vi "Version_2.0_Single_Column_Code.vi"() -> ()   [LabVIEW 2020] (continued)
            n10081 = call "Convert from Dynamic Data6"("Dynamic Data Type"=w10540) -> ("Array"=w10547:dbl[])  [unwired: 3 in]
            n10082 = call-poly <vilib>:"Append Waveforms.vi"("waveform B"=w10545, "waveform A"=w10546) -> ("waveform out"=w10544:waveform(dbl))  [unwired: 8 in, 1 out]
            n10083 = call "Convert from Dynamic Data7"("Dynamic Data Type"=w10544) -> ("Array"=w10548:dbl[])  [unwired: 3 in]
            n10084 = Bundle("Array"=w10547, "Array"=w10548) -> (→"Amplified Signal with Fluid Volume for SEC":cluster{"Array":dbl[], "Array":dbl[]})  [unwired: 1 in]
          }
        }
        n10085 = case shown="True" w10476 {
          tunnel: w10480 -> [w10524 w10531]
          tunnel: w10471 -> [_ w10530]
          tunnel: [w10523 w10529] -> w10478
          tunnel: w10479 -> [w10522 w10527]
          tunnel: [w10521 w10525] -> w10477
          tunnel: w10470 -> [_ w10526]
          frame False {
            n10086 = call-poly <vilib>:"Append Waveforms.vi"("waveform B"=waveform(dbl) {"t0"=timestamp(0 s since 1904-01-01), "dt"=1.0, "Y"=[]}, "waveform A"=w10522) -> ("waveform out"=w10521:waveform(dbl))  [unwired: 8 in, 1 out]
            n10087 = call-poly <vilib>:"Append Waveforms.vi"("waveform B"=waveform(dbl) {"t0"=timestamp(0 s since 1904-01-01), "dt"=1.0, "Y"=[]}, "waveform A"=w10524) -> ("waveform out"=w10523:waveform(dbl))  [unwired: 8 in, 1 out]
          }
          frame True {
            n10088 = call-poly <vilib>:"Append Waveforms.vi"("waveform B"=w10526, "waveform A"=w10527) -> ("waveform out"=w10525:waveform(dbl))  [unwired: 8 in, 1 out]
            n10089 = call "Convert from Dynamic Data10"("Dynamic Data Type"=w10525) -> ("Array"=w10532:dbl[])  [unwired: 3 in]
            n10090 = call-poly <vilib>:"Append Waveforms.vi"("waveform B"=w10530, "waveform A"=w10531) -> ("waveform out"=w10529:waveform(dbl))  [unwired: 8 in, 1 out]
            n10091 = call "Convert from Dynamic Data11"("Dynamic Data Type"=w10529) -> ("Array"=w10533:dbl[])  [unwired: 3 in]
            n10092 = Bundle("Array"=w10532, "Array"=w10533) -> (→"Amplified Signal with Fluid Volume Near Affinity Elution":cluster{"Array":dbl[], "Array":dbl[]})  [unwired: 1 in]
          }
        }
        n10093 = case shown="True" w10469 {
          tunnel: w10475 -> [w10509 w10516]
          tunnel: w10471 -> [_ w10515]
          tunnel: [w10508 w10514] -> w10473
          tunnel: w10474 -> [w10507 w10512]
          tunnel: [w10506 w10511] -> w10472
          tunnel: w10470 -> [_ w10510]
          frame False {
            n10094 = call-poly <vilib>:"Append Waveforms.vi"("waveform B"=waveform(dbl) {"t0"=timestamp(0 s since 1904-01-01), "dt"=1.0, "Y"=[]}, "waveform A"=w10507) -> ("waveform out"=w10506:waveform(dbl))  [unwired: 8 in, 1 out]
            n10095 = call-poly <vilib>:"Append Waveforms.vi"("waveform B"=waveform(dbl) {"t0"=timestamp(0 s since 1904-01-01), "dt"=1.0, "Y"=[]}, "waveform A"=w10509) -> ("waveform out"=w10508:waveform(dbl))  [unwired: 8 in, 1 out]
          }
          frame True {
            n10096 = call-poly <vilib>:"Append Waveforms.vi"("waveform B"=w10510, "waveform A"=w10512) -> ("waveform out"=w10511:waveform(dbl))  [unwired: 8 in, 1 out]
            n10097 = call "Convert from Dynamic Data8"("Dynamic Data Type"=w10511) -> ("Array"=w10517:dbl[])  [unwired: 3 in]
            n10098 = call-poly <vilib>:"Append Waveforms.vi"("waveform B"=w10515, "waveform A"=w10516) -> ("waveform out"=w10514:waveform(dbl))  [unwired: 8 in, 1 out]
            n10099 = call "Convert from Dynamic Data9"("Dynamic Data Type"=w10514) -> ("Array"=w10518:dbl[])  [unwired: 3 in]
            n10100 = Bundle("Array"=w10517, "Array"=w10518) -> (→"Amplified Signal with Fluid Volume for Affinity Elution":cluster{"Array":dbl[], "Array":dbl[]})  [unwired: 1 in]
          }
        }
        n10101 = call-poly <vilib>:"Append Waveforms.vi"("waveform B"=w10471, "waveform A"=w10503) -> ("waveform out"=w10496:waveform(dbl))  [unwired: 8 in, 1 out]
        n10102 = call "Convert from Dynamic Data3"("Dynamic Data Type"=w10496) -> ("Array"=w10499:dbl[])  [unwired: 3 in]
        n10103 = Bundle("Array"=w10498, "Array"=w10499) -> (→"Amplified Signal with Fluid Volume":cluster{"Array":dbl[], "Array":dbl[]})  [unwired: 1 in]
        n10104 = Wait Until Next ms Multiple(millisecond multiple=u32 400) -> ()  [unwired: 1 out]
      }
      n10105 = call-poly "VISA Configure Serial Port"("VISA resource name"=refnum<visa-resource-name> "COM7", "timeout (10sec)"=u32 1000, "baud rate (9600)"=u32 9600) -> ("VISA resource name out"=w69:refnum<visa-resource-name>, "error out"=w68:errorcluster)  [unwired: 11 in]
      n10106 = call <vilib>:"fgt init.vi"() -> ("error out"=w28:errorcluster)  [unwired: 11 in]
      n10107 = call <vilib>:"fgt init.vi"() -> ("error out"=w18:errorcluster)  [unwired: 11 in]
      n10108 = call <vilib>:"fgt init.vi"() -> ("error out"=w12:errorcluster)  [unwired: 11 in]
      n10109 = call <vilib>:"fgt init.vi"() -> ("error out"=w14:errorcluster)  [unwired: 11 in]
      n10110 = call <vilib>:"fgt init.vi"() -> ("error out"=w20:errorcluster)  [unwired: 11 in]
      n10111 = call <vilib>:"fgt init.vi"() -> ("error out"=w16:errorcluster)  [unwired: 11 in]
      n10112 = call <vilib>:"fgt init.vi"() -> ("error out"=w22:errorcluster)  [unwired: 11 in]
      n10113 = call <vilib>:"fgt init.vi"() -> ("error out"=w26:errorcluster)  [unwired: 11 in]
      n10114 = call <vilib>:"fgt init.vi"() -> ("error out"=w24:errorcluster)  [unwired: 11 in]
      n10115 = while {
        tunnel: w28 -> [w478]
        tunnel: [w477] -> w27
        tunnel: w26 -> [w476]
        tunnel: [w475] -> w25
        tunnel: w24 -> [w474]
        tunnel: [w473] -> w23
        tunnel: w22 -> [w472]
        tunnel: [w471] -> w21
        tunnel: w20 -> [w470]
        tunnel: [w469] -> w19
        tunnel: w18 -> [w468]
        tunnel: [w467] -> w17
        tunnel: w16 -> [w466]
        tunnel: [w465] -> w15
        tunnel: w14 -> [w464]
        tunnel: [w463] -> w13
        tunnel: w12 -> [w462]
        tunnel: [w461] -> w11
        stop <- w488 stop-if-true
        # "- Controls the 7 on-chip Valves. \n- By default pressure is applied to close them\n- On-chip Valve opening pressure is applied same as the \nsuction pressure for grid deposition on all the valves"
        n10116 = local read "Valve V1 Open"() -> (w508:bool)
        n10117 = local read "Valve V2 Open"() -> (w494:bool)
        n10118 = local read "Valve V3 Open"() -> (w493:bool)
        n10119 = local read "Valve V4 Open"() -> (w492:bool)
        n10120 = local read "Valve V5 Open"() -> (w491:bool)
        n10121 = local read "Valve V6 Open"() -> (w490:bool)
        n10122 = local read "Valve V7 Open"() -> (w489:bool)
        n10123 = Wait (ms)(milliseconds to wait=u32 100) -> ()  [unwired: 1 out]
        n10124 = local read "Valve V8 Open"() -> (w483:bool)
        n10125 = local read "On-Chip Valve \nClosing\nPressure (mbar)"() -> (w486:dbl)
        n10126 = local read "Stopper that ends \nthe main loops"() -> (w488:bool)
        n10127 = case shown="True" w508 {
          tunnel: [1 0 ("position")] -> w507
          frame False {
          }
          frame True {
          }
        }
        n10128 = case shown="True" w494 {
          tunnel: [1 0 ("position")] -> w505
          frame False {
          }
          frame True {
          }
        }
        n10129 = case shown="True" w493 {
          tunnel: [1 0 ("position")] -> w504
          frame False {
          }
          frame True {
          }
        }
        n10130 = case shown="True" w492 {
          tunnel: [1 0 ("position")] -> w501
          frame False {
          }
          frame True {
          }
        }
        n10131 = case shown="True" w491 {
          tunnel: [1 0 ("position")] -> w499
          frame False {
          }
          frame True {
          }
        }
        n10132 = case shown="True" w490 {
          tunnel: [1 0 ("position")] -> w497
          frame False {
          }
          frame True {
          }
        }
        n10133 = call <vilib>:"fgt set pressure.vi"("error in (no error)"=w478, "pressure"=w486, "pressureIndex"=0 ("module")) -> ("error out"=w477:errorcluster)  [unwired: 8 in]
        n10134 = call <vilib>:"fgt get pressure.vi"("pressureIndex"=u32 1) -> ("pressure out"=w481:sgl)  [unwired: 9 in, 1 out]
        n10135 = call <vilib>:"fgt get pressure.vi"("pressureIndex"=u32 0) -> ("pressure out"=w479:sgl)  [unwired: 9 in, 1 out]
        n10136 = case shown="True" w489 {
          tunnel: [1 0 ("position")] -> w495
          frame False {
          }
          frame True {
          }
        }
        n10137 = case shown="True" w483 {
          tunnel: [1 0 ("position")] -> w484
          frame False {
          }
          frame True {
          }
        }
        n10138 = call <vilib>:"fgt set valve position.vi"("error in (no error)"=w462, "position"=w507, "valveIndex"=u32 0) -> ("error out"=w461:errorcluster)  [unwired: 8 in]
        n10139 = call <vilib>:"fgt set valve position.vi"("error in (no error)"=w464, "position"=w505, "valveIndex"=u32 1) -> ("error out"=w463:errorcluster)  [unwired: 8 in]
        n10140 = call <vilib>:"fgt set valve position.vi"("error in (no error)"=w466, "position"=w504, "valveIndex"=u32 2) -> ("error out"=w465:errorcluster)  [unwired: 8 in]
        n10141 = call <vilib>:"fgt set valve position.vi"("error in (no error)"=w468, "position"=w501, "valveIndex"=u32 3) -> ("error out"=w467:errorcluster)  [unwired: 8 in]
        n10142 = call <vilib>:"fgt set valve position.vi"("error in (no error)"=w470, "position"=w499, "valveIndex"=u32 4) -> ("error out"=w469:errorcluster)  [unwired: 8 in]
        n10143 = call <vilib>:"fgt set valve position.vi"("error in (no error)"=w472, "position"=w497, "valveIndex"=u32 5) -> ("error out"=w471:errorcluster)  [unwired: 8 in]
        n10144 = local write "Valve Closing \nPressure Measured"(w479) -> ()
        n10145 = call <vilib>:"fgt set valve position.vi"("error in (no error)"=w474, "position"=w495, "valveIndex"=u32 6) -> ("error out"=w473:errorcluster)  [unwired: 8 in]
        n10146 = call <vilib>:"fgt set valve position.vi"("error in (no error)"=w476, "position"=w484, "valveIndex"=u32 7) -> ("error out"=w475:errorcluster)  [unwired: 8 in]
        n10147 = local write "Suction pressure \nmeasured"(w481) -> ()
      }
      n10148 = call <vilib>:"fgt close.vi"("error in (no error)"=w27) -> ()  [unwired: 10 in, 1 out]
      n10149 = call <vilib>:"fgt close.vi"("error in (no error)"=w17) -> ()  [unwired: 10 in, 1 out]
      n10150 = call <vilib>:"fgt close.vi"("error in (no error)"=w11) -> ()  [unwired: 10 in, 1 out]
      n10151 = call <vilib>:"fgt close.vi"("error in (no error)"=w13) -> ()  [unwired: 10 in, 1 out]
      n10152 = call <vilib>:"fgt close.vi"("error in (no error)"=w19) -> ()  [unwired: 10 in, 1 out]
      n10153 = call <vilib>:"fgt close.vi"("error in (no error)"=w15) -> ()  [unwired: 10 in, 1 out]
      n10154 = call <vilib>:"fgt close.vi"("error in (no error)"=w21) -> ()  [unwired: 10 in, 1 out]
      n10155 = call <vilib>:"fgt close.vi"("error in (no error)"=w25) -> ()  [unwired: 10 in, 1 out]
      n10156 = call <vilib>:"fgt close.vi"("error in (no error)"=w23) -> ()  [unwired: 10 in, 1 out]
      n10157 = while {
        stop <- w98 stop-if-true
        n10158 = event shown="[2] \"Stop for End of  Experiment  and Data Writing\": Value Change" {
          selector: _ -> [_ _ _]
          dyn-events: _ -> [_ _ _]
          timeout: 100 -> [_ _ _]
          tunnel: [_ _ w105] -> w98
          event Timeout {
            n10159 = event-data() -> ()  [unwired: 1 in, 3 out]
          }
          event "External Valve \nOpen": Value Change {
            n10160 = event-data() -> ()  [unwired: 1 in, 6 out]
            n10161 = local read "External Valve \nOpen"() -> (w100:bool)
            n10162 = case shown="False" w100 {
              frame False {
                # "external vale is closed"
                n10163 = local read "VISA Refnum in\nfor Valve"() -> (w102:refnum<visa-resource-name>)
                n10164 = call "PortChanger_Valve (SubVI).vi"("Port Number"="2", "VISA Refnum in"=w102) -> ()  [unwired: 10 in]
              }
              frame True {
                # "External valve is open"
                n10165 = local read "VISA Refnum in\nfor Valve"() -> (w104:refnum<visa-resource-name>)
                n10166 = call "PortChanger_Valve (SubVI).vi"("Port Number"="1", "VISA Refnum in"=w104) -> ()  [unwired: 10 in]
              }
            }
          }
          event "Stop for End of \nExperiment \nand Data Writing": Value Change {
            n10167 = event-data() -> ()  [unwired: 1 in, 6 out]
            n10168 = local read "Stop for End of \nExperiment \nand Data Writing"() -> (w105:bool)
          }
        }
      }
      n10169 = while {
        tunnel: [w120] -> w71
        tunnel: [w122] -> w70
        tunnel: w69 -> [w133]
        tunnel: w68 -> [w132]
        shift-right: [w121] -> _
        shift-left: w72 -> [w131]
        tunnel: [w130] -> w83
        tunnel: [w129] -> w84
        tunnel: w85 -> [w114]
        tunnel: [w114] -> w86
        tunnel: w10 -> [w112]
        tunnel: w9 -> [w113]
        stop <- w115 stop-if-true
        n10170 = local write "Position"(0 ("Position")) -> ()
        n10171 = local write "k1"(0.0 ("k1")) -> ()
        n10172 = local write "k2"(0.0 ("k2")) -> ()
        n10173 = event shown="[0] \"Select the Action\": Value Change" {
          selector: _ -> [_ _ _ _ _ _ _ _ _ _]
          dyn-events: _ -> [_ _ _ _ _ _ _ _ _ _]
          timeout: 100 -> [_ _ _ _ _ _ _ _ _ _]
          tunnel: w133 -> [w160 w410 w420 w431 w434 w439 w444 w449 w453 w460]
          tunnel: w132 -> [w159 w409 w419 w430 w435 w440 w445 w450 w452 w459]
          tunnel: w131 -> [_ _ _ _ _ _ _ _ _ _]
          tunnel: w112 -> [_ _ _ _ _ _ _ _ w455 w458]
          tunnel: w113 -> [_ _ _ _ _ _ _ _ w454 w457]
          tunnel: [w156 w407 w417 w427 _ _ _ _ w454 w457] -> w130
          tunnel: [w155 _ _ _ _ _ _ _ w455 w458] -> w129
          tunnel: [_ _ _ _ _ _ _ _ w456 _] -> w115
          tunnel: [w158 w408 w418 w428 w432 w437 w442 w447 w453 w460] -> w124
          tunnel: [w157 _ _ _ w433 w438 w443 w448 w452 w459] -> w123
          tunnel: w112 -> [w152 _ _ _ _ _ _ _ _ _]
          tunnel: w113 -> [w153 _ _ _ _ _ _ _ _ _]
          event "Select the Action": Value Change {
            n10174 = event-data() -> ()  [unwired: 1 in, 6 out]
            n10175 = local read "Select the Action"() -> (w154:T1)
            n10176 = case shown="\"Spread the deposited protein on the grid in One Line and plunge\"" w154 {
              tunnel: [w167 w174 w182 w266 w289 w377] -> w158
              tunnel: [w166 w173 w181 w265 w288 w376] -> w157
              tunnel: w160 -> [w165 w172 w180 w270 w287 w375]
              tunnel: w159 -> [w164 w171 w179 w269 w286 w374]
              tunnel: w152 -> [w161 w168 w178 w267 w285 w373]
              tunnel: w153 -> [w162 w169 w177 w268 w284 w372]
              tunnel: [w162 w169 w175 w268 w282 w372] -> w156
              tunnel: [w161 w168 w176 w267 w283 w373] -> w155
              frame .."Turn off Stepper Motor" {
                n10177 = VISA Write(VISA resource name=w165, write buffer="f", error in (no error)=w164) -> (VISA resource name out=w167:refnum<visa-resource-name>, error out=w166:errorcluster)  [unwired: 1 out]
              }
              frame "Turn  on Stepper Motor" {
                n10178 = VISA Write(VISA resource name=w172, write buffer="n", error in (no error)=w171) -> (VISA resource name out=w174:refnum<visa-resource-name>, error out=w173:errorcluster)  [unwired: 1 out]
              }
              frame "Start Plunging" {
                n10179 = stacked-sequence {
                  seq-local: [_ _ _ _ _ w204 _] -> [_ _ _ _ _ _ w263]
                  seq-local: [_ _ _ _ _ w203 _] -> [_ _ _ _ _ _ w262]
                  seq-local: [w184 _ _ _ _ _ _] -> [_ w191 _ _ _ _ _]
                  seq-local: [w183 _ _ _ _ _ _] -> [_ w190 _ _ _ _ _]
                  seq-local: [_ w189 _ _ _ _ _] -> [_ _ _ _ _ w202 _]
                  seq-local: [_ w188 _ _ _ _ _] -> [_ _ _ _ _ w201 _]
                  tunnel: [_ _ _ _ _ _ w261] -> w182
                  tunnel: [_ _ _ _ _ _ w260] -> w181
                  tunnel: w180 -> [_ _ _ _ _ w206 _]
                  tunnel: w179 -> [_ _ _ _ _ w205 _]
                  tunnel: w178 -> [w185 _ _ _ _ _ _]
                  tunnel: w177 -> [w186 _ _ _ _ _ _]
                  tunnel: [_ _ _ _ _ w200 _] -> w176
                  tunnel: [_ _ _ _ _ w199 _] -> w175
                  frame #0 {
                    w187 = 1 items=["Channel1"=1, "Channel2"=2, "Channel3"=3, "Channel4"=4] ("channel")
                    n10180 = invoke class="KCubeInertialMotor" method="SetPositionToZero"(reference=w185, error in=w186, "channel"=w187) -> (reference out=w184:refnum<k24>, error out=w183:errorcluster)  [unwired: 1 in, 2 out]
                  }
                  frame #1 {
                    w192 = 2 items=["Channel1"=1, "Channel2"=2, "Channel3"=3, "Channel4"=4] ("channel")
                    n10181 = invoke class="KCubeInertialMotor" method="SetPositionToZero"(reference=w191, error in=w190, "channel"=w192) -> (reference out=w189:refnum<k24>, error out=w188:errorcluster)  [unwired: 1 in, 2 out]
                  }
                  frame #2 {
                    n10182 = local write "Re-deposit Sample\nonto Grid"(FALSE ("Re-deposit Sample\nonto Grid")) -> ()
                    n10183 = local write "Divert Sample \nonto Grid"(TRUE ("Divert Sample \nonto Grid")) -> ()
                    n10184 = local read "Grid Deposition\nDuration"() -> (w193:u32)
                    n10185 = Wait (ms)(milliseconds to wait=w193) -> ()  [unwired: 1 out]
                  }
                  frame #3 {
                    n10186 = local write "Suction On/Off"(TRUE ("Suction On/Off")) -> ()
                  }
                  frame #4 {
                    n10187 = local read "Delay before\n1st movement\nof grid"() -> (w197:dbl)
                    n10188 = Wait (ms)(milliseconds to wait=w197) -> ()  [unwired: 1 out]
                  }
                  frame #5 {
                    n10189 = local read "No of cycles\nof up-down\nmovement"() -> (w198:dbl)
                    n10190 = for {
                      N: w198 -> [_]
                      shift-right: [w212] -> w204
                      shift-left: w206 -> [w214]
                      shift-right: [w211] -> w203
                      shift-left: w205 -> [w213]
                      shift-right: [w208] -> w200
                      shift-left: w202 -> [w210]
                      shift-right: [w207] -> w199
                      shift-left: w201 -> [w209]
                      n10191 = stacked-sequence {
                        seq-local: [w216 _ _ _ _ _] -> [_ _ _ w238 _ _]
                        seq-local: [w215 _ _ _ _ _] -> [_ _ _ w237 _ _]
                        seq-local: [_ _ w222 _ _ _] -> [_ _ _ _ _ w246]
                        seq-local: [_ _ w221 _ _ _] -> [_ _ _ _ _ w245]
                        tunnel: [_ _ _ w239 _ _] -> w212
                        tunnel: [_ _ _ w241 _ _] -> w211
                        tunnel: w214 -> [w219 _ _ _ _ _]
                        tunnel: w213 -> [w218 _ _ _ _ _]
                        tunnel: w210 -> [_ _ w224 _ _ _]
                        tunnel: w209 -> [_ _ w223 _ _ _]
                        tunnel: [_ _ _ _ _ w244] -> w208
                        tunnel: [_ _ _ _ _ w243] -> w207
                        frame #0 {
                          n10192 = VISA Write(VISA resource name=w219, write buffer="d", error in (no error)=w218) -> (VISA resource name out=w216:refnum<visa-resource-name>, error out=w215:errorcluster)  [unwired: 1 out]
                        }
                        frame #1 {
                          n10193 = local read "Duration for \nup/down\nMovement of Grid"() -> (w220:u32)
                          n10194 = Wait (ms)(milliseconds to wait=w220) -> ()  [unwired: 1 out]
                        }
                        frame #2 {
                          n10195 = stacked-sequence {
                            tunnel: w224 -> [_ w232 _]
                            tunnel: w223 -> [_ w231 _]
                            tunnel: [_ w230 _] -> w222
                            tunnel: [_ w229 _] -> w221
                            frame #0 {
                              n10196 = local read "Translation Step SIze\nwhile plunging"() -> (w225:dbl)
                              n10197 = local read "k1"() -> (w227:dbl)
                              n10198 = Decrement(x=w227) -> (x-1=w226:dbl)
                              n10199 = Multiply(x=w225, y=w226) -> (x*y=w228:dbl)
                              n10200 = local write "k2"(w226) -> ()
                              n10201 = local write "Position"(w228) -> ()
                            }
                            frame #1 {
                              w235 = 1 items=["Channel1"=1, "Channel2"=2, "Channel3"=3, "Channel4"=4] ("channel")
                              n10202 = local read "Position"() -> (w234:i32)
                              n10203 = invoke class="KCubeInertialMotor" method="MoveTo"(reference=w232, error in=w231, "channel"=w235, "position"=w234, "waitTimeout"=10000) -> (reference out=w230:refnum<k24>, error out=w229:errorcluster)  [unwired: 1 in, 4 out]
                            }
                            frame #2 {
                              n10204 = local read "Wait time for\ntranslation"() -> (w236:u32)
                              n10205 = Wait (ms)(milliseconds to wait=w236) -> ()  [unwired: 1 out]
                            }
                          }
                        }
                        frame #3 {
                          n10206 = VISA Write(VISA resource name=w238, write buffer="u", error in (no error)=w237) -> (VISA resource name out=w239:refnum<visa-resource-name>, error out=w241:errorcluster)  [unwired: 1 out]
                        }
                        frame #4 {
                          n10207 = local read "Duration for \nup/down\nMovement of Grid"() -> (w242:u32)
                          n10208 = Wait (ms)(milliseconds to wait=w242) -> ()  [unwired: 1 out]
                        }
                        frame #5 {
                          n10209 = stacked-sequence {
                            tunnel: w246 -> [_ w254 _]
                            tunnel: w245 -> [_ w253 _]
                            tunnel: [_ w252 _] -> w244
                            tunnel: [_ w251 _] -> w243
                            frame #0 {
                              n10210 = local read "Translation Step SIze\nwhile plunging"() -> (w247:dbl)
                              n10211 = local read "k2"() -> (w249:dbl)
                              n10212 = Increment(x=w249) -> (x+1=w248:dbl)
                              n10213 = Multiply(x=w247, y=w248) -> (x*y=w250:dbl)
                              n10214 = local write "k1"(w248) -> ()
                              n10215 = local write "Position"(w250) -> ()
                            }
                            frame #1 {
                              w257 = 1 items=["Channel1"=1, "Channel2"=2, "Channel3"=3, "Channel4"=4] ("channel")
                              n10216 = local read "Position"() -> (w256:i32)
                              n10217 = invoke class="KCubeInertialMotor" method="MoveTo"(reference=w254, error in=w253, "channel"=w257, "position"=w256, "waitTimeout"=10000) -> (reference out=w252:refnum<k24>, error out=w251:errorcluster)  [unwired: 1 in, 4 out]
                            }
                            frame #2 {
                              n10218 = local read "Wait time for\ntranslation"() -> (w258:u32)
                              n10219 = Wait (ms)(milliseconds to wait=w258) -> ()  [unwired: 1 out]
                            }
                          }
                        }
                      }
                    }
                  }
                  frame #6 {
                    n10220 = VISA Write(VISA resource name=w263, write buffer="p", error in (no error)=w262) -> (VISA resource name out=w261:refnum<visa-resource-name>, error out=w260:errorcluster)  [unwired: 1 out]
                    n10221 = local write "Suction On/Off"(FALSE ("Suction On/Off")) -> ()
                  }
                }
              }
              frame "Reset Plunger" {
                n10222 = stacked-sequence {
                  seq-local: [w272 _] -> [_ w280]
                  seq-local: [w271 _] -> [_ w279]
                  tunnel: w270 -> [w276 _]
                  tunnel: w269 -> [w275 _]
                  tunnel: [_ w278] -> w266
                  tunnel: [_ w277] -> w265
                  frame #0 {
                    n10223 = VISA Write(VISA resource name=w276, write buffer="r", error in (no error)=w275) -> (VISA resource name out=w272:refnum<visa-resource-name>, error out=w271:errorcluster)  [unwired: 1 out]
                    n10224 = Wait (ms)(milliseconds to wait=u32 1000) -> ()  [unwired: 1 out]
                  }
                  frame #1 {
                    n10225 = VISA Write(VISA resource name=w280, write buffer="f", error in (no error)=w279) -> (VISA resource name out=w278:refnum<visa-resource-name>, error out=w277:errorcluster)  [unwired: 1 out]
                  }
                }
              }
              frame "Spread the deposited protein on the grid and plunge" {
                n10226 = stacked-sequence {
                  seq-local: [_ _ _ _ _ w311 _] -> [_ _ _ _ _ _ w370]
                  seq-local: [_ _ _ _ _ w310 _] -> [_ _ _ _ _ _ w369]
                  seq-local: [w291 _ _ _ _ _ _] -> [_ w298 _ _ _ _ _]
                  seq-local: [w290 _ _ _ _ _ _] -> [_ w297 _ _ _ _ _]
                  seq-local: [_ w296 _ _ _ _ _] -> [_ _ _ _ _ w309 _]
                  seq-local: [_ w295 _ _ _ _ _] -> [_ _ _ _ _ w308 _]
                  tunnel: [_ _ _ _ _ _ w368] -> w289
                  tunnel: [_ _ _ _ _ _ w367] -> w288
                  tunnel: w287 -> [_ _ _ _ _ w313 _]
                  tunnel: w286 -> [_ _ _ _ _ w312 _]
                  tunnel: w285 -> [w292 _ _ _ _ _ _]
                  tunnel: w284 -> [w293 _ _ _ _ _ _]
                  tunnel: [_ _ _ _ _ w307 _] -> w283
                  tunnel: [_ _ _ _ _ w306 _] -> w282
                  frame #0 {
                    w294 = 1 items=["Channel1"=1, "Channel2"=2, "Channel3"=3, "Channel4"=4] ("channel")
                    n10227 = invoke class="KCubeInertialMotor" method="SetPositionToZero"(reference=w292, error in=w293, "channel"=w294) -> (reference out=w291:refnum<k24>, error out=w290:errorcluster)  [unwired: 1 in, 2 out]
                  }
                  frame #1 {
                    w299 = 2 items=["Channel1"=1, "Channel2"=2, "Channel3"=3, "Channel4"=4] ("channel")
                    n10228 = invoke class="KCubeInertialMotor" method="SetPositionToZero"(reference=w298, error in=w297, "channel"=w299) -> (reference out=w296:refnum<k24>, error out=w295:errorcluster)  [unwired: 1 in, 2 out]
                  }
                  frame #2 {
                    n10229 = local write "Re-deposit Sample\nonto Grid"(FALSE ("Re-deposit Sample\nonto Grid")) -> ()
                    n10230 = local write "Divert Sample \nonto Grid"(TRUE ("Divert Sample \nonto Grid")) -> ()
                    n10231 = local read "Grid Deposition\nDuration"() -> (w300:u32)
                    n10232 = Wait (ms)(milliseconds to wait=w300) -> ()  [unwired: 1 out]
                  }
                  frame #3 {
                    n10233 = local write "Suction On/Off"(TRUE ("Suction On/Off")) -> ()
                  }
                  frame #4 {
                    n10234 = local read "Delay before\n1st movement\nof grid"() -> (w304:dbl)
                    n10235 = Wait (ms)(milliseconds to wait=w304) -> ()  [unwired: 1 out]
                  }
                  frame #5 {
                    n10236 = local read "No of cycles\nof up-down\nmovement"() -> (w305:dbl)
                    n10237 = for {
                      N: w305 -> [_]
                      shift-right: [w319] -> w311
                      shift-left: w313 -> [w321]
                      shift-right: [w318] -> w310
                      shift-left: w312 -> [w320]
                      shift-right: [w315] -> w307
                      shift-left: w309 -> [w317]
                      shift-right: [w314] -> w306
                      shift-left: w308 -> [w316]
                      n10238 = stacked-sequence {
                        seq-local: [w323 _ _ _ _ _] -> [_ _ _ w345 _ _]
                        seq-local: [w322 _ _ _ _ _] -> [_ _ _ w344 _ _]
                        seq-local: [_ _ w329 _ _ _] -> [_ _ _ _ _ w353]
                        seq-local: [_ _ w328 _ _ _] -> [_ _ _ _ _ w352]
                        tunnel: [_ _ _ w346 _ _] -> w319
                        tunnel: [_ _ _ w348 _ _] -> w318
                        tunnel: w321 -> [w326 _ _ _ _ _]
                        tunnel: w320 -> [w325 _ _ _ _ _]
                        tunnel: w317 -> [_ _ w331 _ _ _]
                        tunnel: w316 -> [_ _ w330 _ _ _]
                        tunnel: [_ _ _ _ _ w351] -> w315
                        tunnel: [_ _ _ _ _ w350] -> w314
                        frame #0 {
                          n10239 = VISA Write(VISA resource name=w326, write buffer="d", error in (no error)=w325) -> (VISA resource name out=w323:refnum<visa-resource-name>, error out=w322:errorcluster)  [unwired: 1 out]
                        }
                        frame #1 {
                          n10240 = local read "Duration for \nup/down\nMovement of Grid"() -> (w327:u32)
                          n10241 = Wait (ms)(milliseconds to wait=w327) -> ()  [unwired: 1 out]
                        }
                        frame #2 {
                          n10242 = stacked-sequence {
                            tunnel: w331 -> [_ w339 _]
                            tunnel: w330 -> [_ w338 _]
                            tunnel: [_ w337 _] -> w329
                            tunnel: [_ w336 _] -> w328
                            frame #0 {
                              n10243 = local read "Translation Step SIze\nwhile plunging"() -> (w332:dbl)
                              n10244 = local read "k1"() -> (w334:dbl)
                              n10245 = Decrement(x=w334) -> (x-1=w333:dbl)
                              n10246 = Multiply(x=w332, y=w333) -> (x*y=w335:dbl)
                              n10247 = local write "k2"(w333) -> ()
                              n10248 = local write "Position"(w335) -> ()
                            }
                            frame #1 {
                              w342 = 1 items=["Channel1"=1, "Channel2"=2, "Channel3"=3, "Channel4"=4] ("channel")
                              n10249 = local read "Position"() -> (w341:i32)
                              n10250 = invoke class="KCubeInertialMotor" method="MoveTo"(reference=w339, error in=w338, "channel"=w342, "position"=w341, "waitTimeout"=10000) -> (reference out=w337:refnum<k24>, error out=w336:errorcluster)  [unwired: 1 in, 4 out]
                            }
                            frame #2 {
                              n10251 = local read "Wait time for\ntranslation"() -> (w343:u32)
                              n10252 = Wait (ms)(milliseconds to wait=w343) -> ()  [unwired: 1 out]
                            }
                          }
                        }
                        frame #3 {
                          n10253 = VISA Write(VISA resource name=w345, write buffer="u", error in (no error)=w344) -> (VISA resource name out=w346:refnum<visa-resource-name>, error out=w348:errorcluster)  [unwired: 1 out]
                        }
                        frame #4 {
                          n10254 = local read "Duration for \nup/down\nMovement of Grid"() -> (w349:u32)
                          n10255 = Wait (ms)(milliseconds to wait=w349) -> ()  [unwired: 1 out]
                        }
                        frame #5 {
                          n10256 = stacked-sequence {
                            tunnel: w353 -> [_ w361 _]
                            tunnel: w352 -> [_ w360 _]
                            tunnel: [_ w359 _] -> w351
                            tunnel: [_ w358 _] -> w350
                            frame #0 {
                              n10257 = local read "Translation Step SIze\nwhile plunging"() -> (w354:dbl)
                              n10258 = local read "k2"() -> (w356:dbl)
                              n10259 = Increment(x=w356) -> (x+1=w355:dbl)
                              n10260 = Multiply(x=w354, y=w355) -> (x*y=w357:dbl)
                              n10261 = local write "k1"(w355) -> ()
                              n10262 = local write "Position"(w357) -> ()
                            }
                            frame #1 {
                              w364 = 1 items=["Channel1"=1, "Channel2"=2, "Channel3"=3, "Channel4"=4] ("channel")
                              n10263 = local read "Position"() -> (w363:i32)
                              n10264 = invoke class="KCubeInertialMotor" method="MoveTo"(reference=w361, error in=w360, "channel"=w364, "position"=w363, "waitTimeout"=10000) -> (reference out=w359:refnum<k24>, error out=w358:errorcluster)  [unwired: 1 in, 4 out]
                            }
                            frame #2 {
                              n10265 = local read "Wait time for\ntranslation"() -> (w365:u32)
                              n10266 = Wait (ms)(milliseconds to wait=w365) -> ()  [unwired: 1 out]
                            }
                          }
                        }
                      }
                    }
                  }
                  frame #6 {
                    n10267 = VISA Write(VISA resource name=w370, write buffer="p", error in (no error)=w369) -> (VISA resource name out=w368:refnum<visa-resource-name>, error out=w367:errorcluster)  [unwired: 1 out]
                    n10268 = local write "Suction On/Off"(FALSE ("Suction On/Off")) -> ()
                  }
                }
              }
              frame "Spread the deposited protein on the grid in One Line and plunge" {
                n10269 = stacked-sequence {
                  seq-local: [_ _ _ w386 _ _] -> [_ _ _ _ w403 _]
                  seq-local: [_ _ _ w385 _ _] -> [_ _ _ _ w402 _]
                  tunnel: [_ _ _ _ w401 _] -> w377
                  tunnel: [_ _ _ _ w400 _] -> w376
                  tunnel: w375 -> [_ _ _ w388 _ _]
                  tunnel: w374 -> [_ _ _ w387 _ _]
                  frame #0 {
                    n10270 = local write "Re-deposit Sample\nonto Grid"(FALSE ("Re-deposit Sample\nonto Grid")) -> ()
                    n10271 = local write "Divert Sample \nonto Grid"(TRUE ("Divert Sample \nonto Grid")) -> ()
                    n10272 = local read "Grid Deposition\nDuration"() -> (w378:u32)
                    n10273 = Wait (ms)(milliseconds to wait=w378) -> ()  [unwired: 1 out]
                  }
                  frame #1 {
                    n10274 = local write "Suction On/Off"(TRUE ("Suction On/Off")) -> ()
                    n10275 = Wait (ms)(milliseconds to wait=u32 50) -> ()  [unwired: 1 out]
                  }
                  frame #2 {
                    n10276 = local read "Delay before\n1st movement\nof grid"() -> (w383:dbl)
                    n10277 = Wait (ms)(milliseconds to wait=w383) -> ()  [unwired: 1 out]
                  }
                  frame #3 {
                    n10278 = local read "No of cycles\nof up-down\nmovement"() -> (w384:dbl)
                    n10279 = for {
                      N: w384 -> [_]
                      shift-right: [w390] -> w386
                      shift-left: w388 -> [w392]
                      shift-right: [w389] -> w385
                      shift-left: w387 -> [w391]
                      n10280 = stacked-sequence {
                        tunnel: w392 -> [w397 _]
                        tunnel: w391 -> [w396 _]
                        tunnel: [w394 _] -> w390
                        tunnel: [w393 _] -> w389
                        frame #0 {
                          n10281 = VISA Write(VISA resource name=w397, write buffer="y", error in (no error)=w396) -> (VISA resource name out=w394:refnum<visa-resource-name>, error out=w393:errorcluster)  [unwired: 1 out]
                        }
                        frame #1 {
                          n10282 = local read "Duration for \nup/down\nMovement of Grid"() -> (w398:u32)
                          n10283 = Wait (ms)(milliseconds to wait=w398) -> ()  [unwired: 1 out]
                        }
                      }
                    }
                  }
                  frame #4 {
                    n10284 = VISA Write(VISA resource name=w403, write buffer="p", error in (no error)=w402) -> (VISA resource name out=w401:refnum<visa-resource-name>, error out=w400:errorcluster)  [unwired: 1 out]
                    n10285 = local write "Suction On/Off"(FALSE ("Suction On/Off")) -> ()
                  }
                  frame #5 {
                    n10286 = local write "Suction On/Off"(FALSE ("Suction On/Off")) -> ()
                    n10287 = Wait (ms)(milliseconds to wait=u32 50) -> ()  [unwired: 1 out]
                  }
                }
              }
            }
          }
          event "Set - Blotting Time": Value Change {
            n10288 = event-data() -> ()  [unwired: 1 in, 6 out]
            n10289 = local read "Blotting Time"() -> (w414:dbl)
            n10290 = Format Into String(format string="%0d", w414) -> (resulting string=w413:string)  [unwired: 2 in, 1 out]
            n10291 = Concatenate Strings("t" ("string"), w413, "\r\n") -> (w411:string)
            n10292 = VISA Write(VISA resource name=w410, write buffer=w411, error in (no error)=w409) -> (VISA resource name out=w408:refnum<visa-resource-name>, error out=w407:errorcluster)  [unwired: 1 out]
          }
          event "Set - Blotting Angle": Value Change {
            n10293 = event-data() -> ()  [unwired: 1 in, 6 out]
            n10294 = local read "Blotting Angle"() -> (w424:dbl)
            n10295 = Format Into String(format string="%0d", w424) -> (resulting string=w423:string)  [unwired: 2 in, 1 out]
            n10296 = Concatenate Strings("b" ("string"), w423, "\r\n") -> (w421:string)
            n10297 = VISA Write(VISA resource name=w420, write buffer=w421, error in (no error)=w419) -> (VISA resource name out=w418:refnum<visa-resource-name>, error out=w417:errorcluster)  [unwired: 1 out]
          }
          event "Automated Blotting \nand Plunging": Value Change {
            n10298 = event-data() -> ()  [unwired: 1 in, 6 out]
            n10299 = VISA Write(VISA resource name=w431, write buffer="z", error in (no error)=w430) -> (VISA resource name out=w428:refnum<visa-resource-name>, error out=w427:errorcluster)  [unwired: 1 out]
          }
          event "Move\nGrid Up": Value Change {
            n10300 = event-data() -> ()  [unwired: 1 in, 6 out]
            n10301 = VISA Write(VISA resource name=w434, write buffer="h", error in (no error)=w435) -> (VISA resource name out=w432:refnum<visa-resource-name>, error out=w433:errorcluster)  [unwired: 1 out]
          }
          event "Move Grid \nUp Faster": Value Change {
            n10302 = event-data() -> ()  [unwired: 1 in, 6 out]
            n10303 = VISA Write(VISA resource name=w439, write buffer="x", error in (no error)=w440) -> (VISA resource name out=w437:refnum<visa-resource-name>, error out=w438:errorcluster)  [unwired: 1 out]
          }
          event "Move\nGrid Down": Value Change {
            n10304 = event-data() -> ()  [unwired: 1 in, 6 out]
            n10305 = VISA Write(VISA resource name=w444, write buffer="l", error in (no error)=w445) -> (VISA resource name out=w442:refnum<visa-resource-name>, error out=w443:errorcluster)  [unwired: 1 out]
          }
          event "Move Grid \nDown Faster": Value Change {
            n10306 = event-data() -> ()  [unwired: 1 in, 6 out]
            n10307 = VISA Write(VISA resource name=w449, write buffer="y", error in (no error)=w450) -> (VISA resource name out=w447:refnum<visa-resource-name>, error out=w448:errorcluster)  [unwired: 1 out]
          }
          event "Stop for End of \nExperiment \nand Data Writing": Value Change {
            n10308 = event-data() -> ()  [unwired: 1 in, 6 out]
            n10309 = local read "Stop for End of \nExperiment \nand Data Writing"() -> (w456:bool)
          }
          event Timeout {
            n10310 = event-data() -> ()  [unwired: 1 in, 3 out]
          }
        }
        n10311 = property class="Instr"(reference=w124, error in=w123) -> (reference out=w125:refnum<visa-resource-name>, error out=w126:errorcluster, "Serial Settings:Number of Bytes at Serial Port"=w128:u32)
        n10312 = Greater Than 0?(x=w128) -> (x > 0?=w127:bool)
        n10313 = case shown="True" w127 {
          tunnel: [w136 w151] -> w120
          tunnel: [w135 w150] -> w122
          tunnel: w125 -> [w136 w148]
          tunnel: w126 -> [w135 w147]
          tunnel: [w134 w146] -> w121
          tunnel: w131 -> [w134 w145]
          frame False {
          }
          frame True {
            (unwired) u32 20 ("byte count")
            n10314 = VISA Read(VISA resource name=w148, byte count=16, error in (no error)=w147) -> (VISA resource name out=w151:refnum<visa-resource-name>, read buffer=w144:string, error out=w150:errorcluster)  [unwired: 1 out]
            n10315 = Spreadsheet String To Array(delimiter (Tab)=",", format string="%f", spreadsheet string=w144, array type (2D Dbl)=dbl[] []) -> (array=w140:dbl[])
            n10316 = Index Array(array=w140) -> (element #1=w137:dbl, element #2=→"Ethane Temperature":dbl)  [unwired: 2 in]
            "RH (%)" <- w137
            n10317 = call "Convert from Dynamic Data5"("Dynamic Data Type"=w137) -> ("Array"=w139:dbl[])  [unwired: 3 in]
            n10318 = call-poly <vilib>:"Append Waveforms.vi"("waveform B"=w139, "waveform A"=w145) -> ("waveform out"=w146:waveform(dbl))  [unwired: 8 in, 1 out]
            "Temperature of Ethane Graph" <- w146
          }
        }
      }
      n10319 = Merge Signals(w88, w87) -> (w89:dynamicdata)
      n10320 = call "Write To Measurement File"("Signals"=w89) -> ()  [unwired: 16 in, 3 out]
      n10321 = VISA Close(VISA resource name=w71, error in (no error)=w70) -> ()  [unwired: 1 out]
      n10322 = invoke class="KCubeInertialMotor" method="StopPolling"(reference=w84, error in=w83) -> (error out=w82:errorcluster)  [unwired: 1 in, 2 out]
      n10323 = invoke class="KCubeInertialMotorControl" method="CloseDevice"(reference=w86, error in=w82) -> ()  [unwired: 1 in, 3 out]
      "Discard fluid \nprior to 1st \ndeposition" <- FALSE ("Discard fluid \nprior to 1st \ndeposition")
      "SEC On" <- FALSE ("SEC On")
      "Affinity On" <- FALSE ("Affinity On")
      "Affinity Elution On" <- FALSE ("Affinity On")
      "Suction pressure \nfor grid deposition" <- sgl 0.0 ("Suction pressure \nfor grid deposition")
      "Net Elution \nVolume" <- 0.0 ("Net Elution \nVolume")
      "Pause Elution" <- FALSE ("Pause Elution")
    }
    frame #1 {
      # "Switch off the LEDs"
      n10324 = local write "Start the Process"(FALSE ("Start the Process")) -> ()
      n10325 = local write "Stop for End of \nExperiment \nand Data Writing"(FALSE ("Stop for End of \nExperiment \nand Data Writing")) -> ()
      n10326 = local write "Stopper that ends \nthe main loops"(FALSE ("Stopper that ends \nthe main loops")) -> ()
    }
  }
  "Volume being Injected \nin this process" <- 0.0 ("Volume being Injected \nin this process")
  "Total Volume \nbeing Injected" <- 0.0 ("Total Volume being Injected")
  "Volume being Injected \ntill the end of previous \nprocess" <- 0.0 ("Volume being Injected \ntill the end of previous \nprocess")
  "Pause Data Collection" <- TRUE ("Pause Data Collection")
  "Stopper that ends \nthe main loops" <- FALSE ("Stopper that ends \nthe main loops")
  "Initial Plunger Position" <- 0 ("Initial Plunger Position")
  "True Volume being \ninjected in this\nprocess" <- 0.0
  "Affinity Elution \nis Approaching" <- FALSE ("Affinity Elution \nis Approaching")
